vi "ConnectToDMM.vi"(0 "Min Voltage (V)":dbl, 1 "Max Voltage (V)":dbl, 4 "Step (V)":dbl) -> (14 "VISA resource name out":refnum<visa-resource-name>, 15 "error out":errorcluster, 16 "Min Voltage (V) 2":dbl, 17 "Step (V) 2":dbl, 18 "Current_Date":string caption="Datum mìøení", 19 "unsigned 64bit integer":u64)   [LabVIEW 2021]
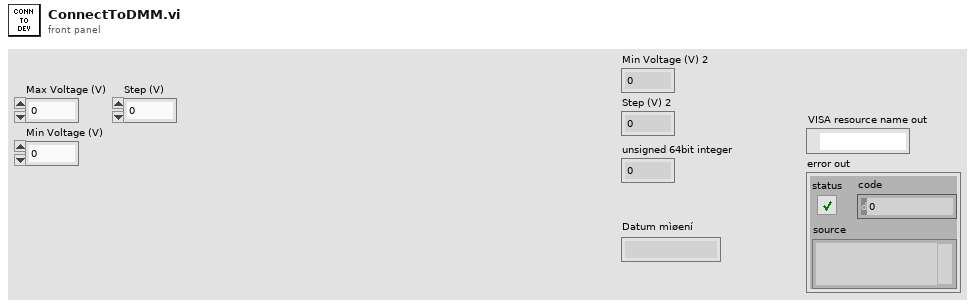
[diagram p1: front panel]
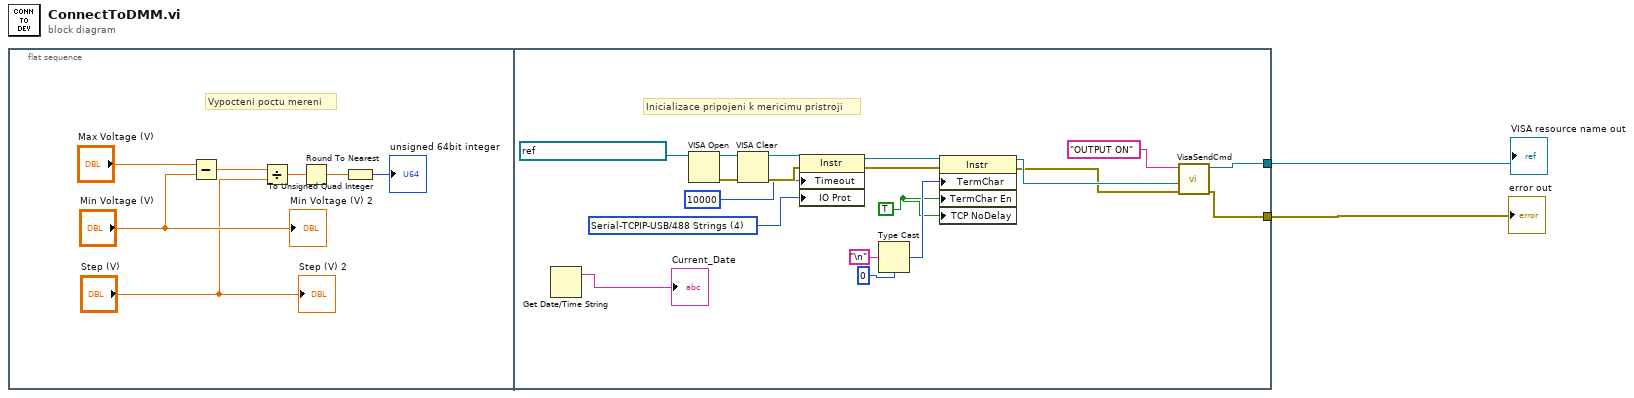
[diagram p0: block diagram]
diagram:
  n1 = flat-sequence {
    tunnel: [w26] -> w2
    tunnel: [w25] -> w1
    frame #0 {
      # "Vypocteni poctu mereni"
      n2 = Subtract(x="Max Voltage (V)", y="Min Voltage (V)") -> (x-y=w7:dbl)
      n3 = Divide(x=w7, y="Step (V)") -> (x/y=w5:dbl)
      n4 = Round To Nearest(number=w5) -> (nearest integer value=w4:dbl)
      n5 = To Unsigned Quad Integer(1:w4) -> (0:→"unsigned 64bit integer":u64)
      "Min Voltage (V) 2" <- "Min Voltage (V)"
      "Step (V) 2" <- "Step (V)"
    }
    frame #1 {
      w12 = TRUE
      w18 = u16 4 items=["Normal"=1, "VXI/FDC"=2, "GPIB/HS488"=3, "Serial-TCPIP-USB/488 Strings"=4, "USBTMC/Vendor-Specific"=5] ("Message Based Settings:IO Protocol")
      # "Inicializace pripojeni k mericimu pristroji"
      n6 = Get Date/Time String() -> (date string=→"Current_Date":string)  [unwired: 3 in, 1 out]
      n7 = VISA Open(VISA resource name=refnum<visa-resource-name> "DMMandPowerSupply") -> (VISA resource name=w22:refnum<visa-resource-name>, error out=w23:errorcluster)  [unwired: 4 in]
      n8 = VISA Clear(VISA resource name=w22, error in (no error)=w23) -> (VISA resource name out=w21:refnum<visa-resource-name>, error out=w20:errorcluster)
      n9 = property class="Instr"(reference=w21, error in=w20, "Timeout"=u32 10000 ("General Settings:Timeout Value"), "IO Prot"=w18) -> (reference out=w17:refnum<visa-resource-name>, error out=w16:errorcluster)
      n10 = Type Cast(type=u8 0, x="\n" ("Line Feed Constant")) -> (*(type *) &x=w13:u8)
      n11 = property class="Instr"(reference=w17, error in=w16, "TermChar"=w13, "TermChar En"=w12, "TCP NoDelay"=w12) -> (reference out=w11:refnum<visa-resource-name>, error out=w10:errorcluster)
      n12 = call "VisaSendCmd.vi"("error in (no error)"=w10, "VISA resource name"=w11, "Msg to send"="OUTPUT ON") -> ("error out"=w25:errorcluster, "VISA resource output"=w26:refnum<visa-resource-name>)  [unwired: 7 in]
    }
  }
  "VISA resource name out" <- w2
  "error out" <- w1
